vi "GET_AC_IR DATA.vi"(8 "error in (no error)":errorcluster caption="错误输入（无错误）", 10 "IR_SET DATA":string[](array[string]), 11 "AC_SET DATA":string[](array[string])) -> (0 "error out":errorcluster caption="错误输出", 2 "IR SET DATA OUT":string[](array[string]), 3 "AC SET DATA OUT":string[](array[string]))   [LabVIEW 2018]
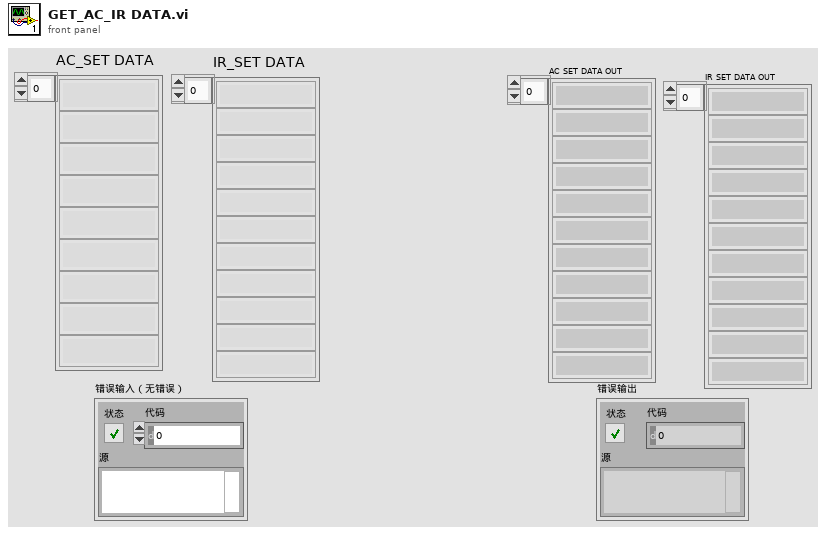
[diagram p1: front panel]
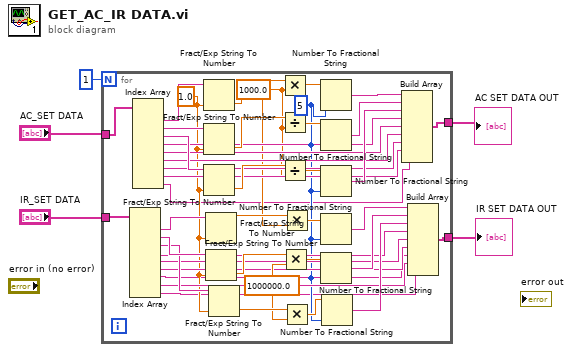
[diagram p0: block diagram]
diagram:
  n1 = for {
    N: 1 -> [_]
    tunnel: "IR_SET DATA" -> [w24]
    tunnel: "AC_SET DATA" -> [w37]
    tunnel: [w36] -> w5
    tunnel: [w26] -> w2
    w17 = 1000000.0 ("y")
    w8 = i16 5 ("精度(6)")
    w27 = 1000.0 ("y")
    w10 = 1.0 ("默认(0 DBL)")
    n2 = Index Array(array=w24) -> (element #1=w23:string, element #2=w22:string, element #3=w19:string, element #4=w14:string, element #5=w13:string, element #6=w12:string, element #7=w9:string, element #8=w11:string, element #9=w6:string)  [unwired: 9 in]
    n3 = Index Array(array=w37) -> (element #1=w45:string, element #2=w35:string, element #3=w34:string, element #4=w33:string, element #5=w32:string, element #6=w31:string, element #7=w30:string, element #8=w29:string, element #9=w7:string)  [unwired: 9 in]
    n4 = Fract/Exp String To Number(string=w45, default (0 dbl)=w10) -> (number=w49:dbl)  [unwired: 2 in, 1 out]
    n5 = Fract/Exp String To Number(string=w35, default (0 dbl)=w10) -> (number=w41:dbl)  [unwired: 2 in, 1 out]
    n6 = Fract/Exp String To Number(string=w34, default (0 dbl)=w10) -> (number=w39:dbl)  [unwired: 2 in, 1 out]
    n7 = Fract/Exp String To Number(string=w23, default (0 dbl)=w10) -> (number=w48:dbl)  [unwired: 2 in, 1 out]
    n8 = Fract/Exp String To Number(string=w22, default (0 dbl)=w10) -> (number=w20:dbl)  [unwired: 2 in, 1 out]
    n9 = Fract/Exp String To Number(string=w19, default (0 dbl)=w10) -> (number=w18:dbl)  [unwired: 2 in, 1 out]
    n10 = Multiply(x=w49, y=w27) -> (x*y=w47:dbl)
    n11 = Divide(x=w41, y=w27) -> (x/y=w42:dbl)
    n12 = Divide(x=w39, y=w27) -> (x/y=w40:dbl)
    n13 = Multiply(x=w20, y=w17) -> (x*y=w25:dbl)
    n14 = Multiply(x=w48, y=w27) -> (x*y=w46:dbl)
    n15 = Multiply(x=w18, y=w17) -> (x*y=w16:dbl)
    n16 = Number To Fractional String(number=w47, precision (6)=w8) -> (F-format string=w44:string)  [unwired: 2 in]
    n17 = Number To Fractional String(number=w42, precision (6)=w8) -> (F-format string=w43:string)  [unwired: 2 in]
    n18 = Number To Fractional String(number=w40, precision (6)=w8) -> (F-format string=w38:string)  [unwired: 2 in]
    n19 = Number To Fractional String(number=w46, precision (6)=w8) -> (F-format string=w28:string)  [unwired: 2 in]
    n20 = Number To Fractional String(number=w25, precision (6)=w8) -> (F-format string=w21:string)  [unwired: 2 in]
    n21 = Number To Fractional String(number=w16, precision (6)=w8) -> (F-format string=w15:string)  [unwired: 2 in]
    n22 = Build Array(w44, w43, w38, w33, w32, w31, w30, w29, w7) -> (w36:string[])
    n23 = Build Array(w28, w21, w15, w14, w13, w12, w9, w11, w6) -> (w26:string[])
  }
  "AC SET DATA OUT" <- w5
  "IR SET DATA OUT" <- w2
